vi "Scott -- strain -- plot staff V0.vi"(8 "error IN":errorcluster, 10 "plots control":cluster{"data string in":string, bool, bool}[](array[cluster]), 11 "data":dbl[][](array[numeric])) -> (0 "error out":errorcluster, 1 "Lockin 1 Graph":cluster{"X Data":dbl[], "Y Data":dbl[]}[](graph)=[{"X Data"=array[300 elements], "Y Data"=array[300 elements]}, {"X Data"=array[300 elements], "Y Data"=[0.34598, 0.34601, 0.34601, 0.34598, 0.34598, 0.34598, 0.34598, 0.34598, 0.34598, 0.34598, 0.34598, 0.34598, 0.34598, 0.345949, 0.34598, 0.34598, 0.34598, 0.34598, 0.34598, 0.34598, 0.34598, 0.34598, 0.34598, 0.34598, 0.34598, 0.34598, 0.34598, 0.34598, 0.34598, 0.34598, 0.34598, 0.34598, 0.34598, 0.34601, 0.34601, 0.34601, 0.34601, 0.34601, 0.34601, 0.34601, 0.34601, 0.34601, 0.34601, 0.34601, 0.34601, 0.34601, 0.34601, 0.346041, 0.346041, 0.346041, 0.346041, 0.346041, 0.346041, 0.346041, 0.346041, 0.346071, 0.346071, 0.346071, 0.346071, 0.346071, 0.346071, 0.346071, 0.346071, 0.346071, 0.346071, 0.346071, 0.346071, 0.346071, 0.346071, 0.346071, 0.346071, 0.346071, 0.346071, 0.346071, 0.346041, 0.346071, 0.346071, 0.346071, 0.346041, 0.346041, 0.346041, 0.346041, 0.346041, 0.34601, 0.346041, 0.346041, 0.34601, 0.34601, 0.34601, 0.34601, 0.34601, 0.34601, 0.34601, 0.34601, 0.34601, 0.34601, 0.34601, 0.34601, 0.34601, 0.34598, 0.34598, 0.34598, 0.34601, 0.34598, 0.34598, 0.34598, 0.34598, 0.34598, 0.34598, 0.34598, 0.34598, 0.34598, 0.34598, 0.34598, 0.34598, 0.34598, 0.34598, 0.34598, 0.34598, 0.34598, 0.34598, 0.34598, 0.34598, 0.34598, 0.34598, 0.34598, 0.34598, 0.34598, 0.34598, 0.34598, 0.34598, 0.34598, 0.34598, 0.34601, 0.34601, 0.34601, 0.34601, 0.34601, 0.34601, 0.34601, 0.34601, 0.34601, 0.34601, 0.34601, 0.34601, 0.34601, 0.346041, 0.346041, 0.34601, 0.34601, 0.346041, 0.346041, 0.346041, 0.346041, 0.346041, 0.346071, 0.346071, 0.346041, 0.346071, 0.346071, 0.346071, 0.346071, 0.346071, 0.346071, 0.346071, 0.346071, 0.346071, 0.346071, 0.346071, 0.346071, 0.346071, 0.346071, 0.346041, 0.346041, 0.346071, 0.346041, 0.346041, 0.346041, 0.346041, 0.346041, 0.346041, 0.34601, 0.346041, 0.346041, 0.34601, 0.34601, 0.34601, 0.34601, 0.34601, 0.34601, 0.34601, 0.34601, 0.34601, 0.34601, 0.34601, 0.34601, 0.34601, 0.34601, 0.34598, 0.34598, 0.34598, 0.34598, 0.34598, 0.34598, 0.34598, 0.34598, 0.34598, 0.34598, 0.34598, 0.34598, 0.34598, 0.34598, 0.34598, 0.34598, 0.34598, 0.345949, 0.34598, 0.34598, 0.34598, 0.34598, 0.34598, 0.34598, 0.34598, 0.34598, 0.34598, 0.34598, 0.34598, 0.34598, 0.34598, 0.34598, 0.34601, 0.34601, 0.34601, 0.34601, 0.34601, 0.34601, 0.34601, 0.34601, 0.34601, 0.34601, 0.34601, 0.34601, 0.34601, 0.34601, 0.34601, 0.34601, 0.34601, 0.346041, 0.346041, 0.346041, 0.346041, 0.346041, 0.346071, 0.346071, 0.346041, 0.346041, 0.346071, 0.346071, 0.346071, 0.346071, 0.346071, 0.346071, 0.346071, 0.346071, 0.346071, 0.346071, 0.346071, 0.346071, 0.346071, 0.346071, 0.346071, 0.346071, 0.346071, 0.346071, 0.346071, 0.346071, 0.346071, 0.346071, 0.346071, 0.346041, 0.346041, 0.346041, 0.346041, 0.346041, 0.34601, 0.346041, 0.346041, 0.34601, 0.34601, 0.34601, 0.34601, 0.34601, 0.34601, 0.34601, 0.34601, 0.34601, 0.34601, 0.34601, 0.34601, 0.34601]}, {"X Data"=array[300 elements], "Y Data"=array[300 elements]}, {"X Data"=array[300 elements], "Y Data"=[0.018135, 0.018139, 0.018133, 0.018133, 0.018137, 0.018135, 0.018133, 0.018133, 0.018131, 0.018129, 0.018129, 0.018127, 0.018131, 0.018131, 0.018127, 0.018127, 0.018127, 0.018125, 0.018127, 0.018127, 0.018123, 0.018129, 0.018131, 0.018127, 0.018135, 0.018139, 0.018139, 0.01814, 0.01814, 0.018137, 0.018131, 0.018131, 0.018127, 0.018137, 0.01814, 0.018139, 0.018135, 0.018133, 0.018139, 0.018135, 0.018139, 0.018144, 0.018142, 0.01814, 0.018144, 0.01815, 0.018144, 0.018146, 0.01814, 0.018139, 0.018135, 0.018129, 0.018129, 0.018135, 0.018142, 0.01814, 0.01814, 0.018142, 0.018146, 0.018144, 0.018144, 0.01815, 0.018144, 0.01814, 0.01814, 0.018137, 0.018137, 0.018137, 0.01814, 0.01814, 0.018137, 0.018131, 0.018131, 0.018137, 0.018137, 0.018144, 0.01814, 0.018131, 0.018131, 0.018129, 0.018131, 0.018139, 0.018148, 0.018144, 0.018139, 0.018133, 0.018131, 0.018133, 0.018127, 0.018129, 0.018119, 0.018123, 0.018125, 0.018127, 0.018133, 0.018133, 0.018131, 0.018129, 0.018131, 0.018133, 0.018129, 0.018129, 0.018131, 0.018133, 0.018127, 0.018123, 0.018121, 0.018125, 0.018127, 0.018131, 0.018129, 0.018127, 0.018127, 0.018127, 0.018129, 0.018123, 0.018127, 0.018125, 0.018116, 0.018116, 0.018127, 0.018127, 0.018123, 0.018121, 0.018125, 0.018127, 0.018127, 0.018127, 0.018135, 0.018135, 0.018129, 0.018131, 0.018125, 0.018118, 0.018121, 0.018135, 0.018139, 0.01814, 0.018146, 0.018142, 0.01814, 0.018137, 0.018127, 0.018127, 0.018135, 0.01814, 0.01814, 0.018137, 0.018127, 0.018133, 0.018137, 0.018142, 0.018142, 0.01814, 0.01814, 0.01814, 0.018142, 0.01814, 0.018135, 0.01814, 0.01814, 0.018135, 0.018139, 0.018139, 0.01814, 0.01814, 0.018146, 0.018146, 0.01814, 0.018144, 0.018146, 0.018144, 0.018139, 0.018139, 0.018135, 0.018137, 0.01814, 0.01814, 0.018139, 0.018131, 0.018139, 0.018139, 0.018133, 0.018135, 0.018129, 0.018131, 0.018137, 0.018133, 0.018135, 0.018139, 0.018139, 0.018137, 0.018133, 0.018129, 0.018129, 0.018125, 0.018129, 0.018135, 0.018133, 0.018135, 0.018125, 0.018127, 0.018123, 0.018125, 0.018127, 0.018127, 0.018125, 0.018125, 0.018125, 0.018125, 0.018127, 0.018127, 0.018133, 0.018129, 0.018129, 0.018127, 0.018123, 0.018131, 0.018129, 0.018129, 0.018133, 0.018131, 0.018137, 0.018137, 0.018135, 0.018135, 0.018129, 0.018133, 0.018137, 0.018135, 0.018131, 0.018129, 0.018131, 0.018135, 0.018139, 0.01814, 0.018139, 0.018139, 0.018129, 0.018131, 0.01814, 0.018127, 0.018131, 0.018133, 0.018129, 0.018131, 0.018137, 0.018131, 0.018135, 0.01814, 0.018139, 0.018135, 0.018135, 0.018133, 0.018137, 0.018139, 0.018137, 0.018133, 0.01814, 0.01814, 0.018133, 0.018133, 0.018133, 0.01814, 0.018146, 0.018148, 0.018142, 0.01814, 0.01814, 0.018135, 0.018131, 0.01814, 0.01814, 0.01814, 0.01814, 0.01814, 0.018135, 0.018133, 0.018139, 0.018133, 0.018129, 0.018135, 0.018133, 0.018135, 0.018135, 0.018135, 0.018137, 0.018135, 0.018135, 0.018135, 0.018131, 0.018131, 0.018125, 0.018125, 0.018129, 0.018129, 0.018127, 0.018125, 0.018121, 0.018118]}] caption="XY Graph")   [LabVIEW 2014]
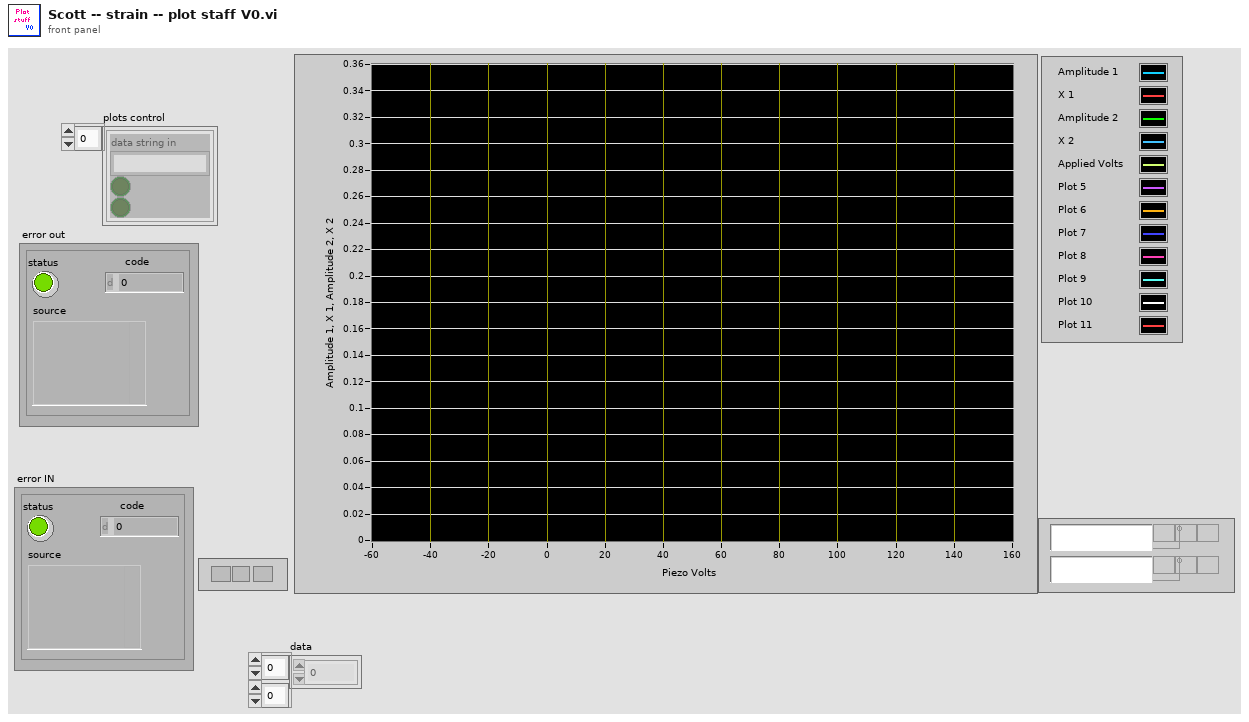
[diagram p1: front panel]
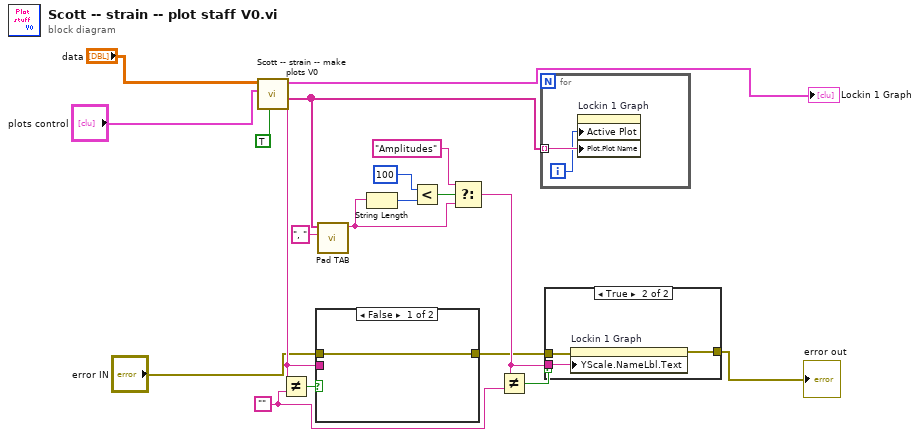
[diagram p0: block diagram]
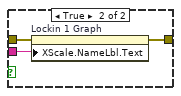
[diagram p3: hidden frame]
diagram:
  w9 = ""
  n1 = call "Scott -- strain -- make plots V0.vi"("transpose? (no:F)"=TRUE, "Channels to plot"="plots control", "Data"="data") -> ("Y-axis names"=w5:string[], "X-axis name"=w8:string, "Plots"=→"Lockin 1 Graph":cluster{"X Data":dbl[], "Y Data":dbl[]}[])  [unwired: 4 in, 2 out]
  n2 = Not Equal?(x=w8, y=w9) -> (x != y?=w11:bool)
  n3 = case shown="False" w11 {
    tunnel: w8 -> [_ w23]
    tunnel: "error IN" -> [w20 w22]
    tunnel: [w20 w21] -> w6
    frame False {
    }
    frame True {
      n4 = property on="Lockin 1 Graph" class="XYGraph (strict)"(error in=w22, "XScale.NameLbl.Text"=w23) -> (error out=w21:errorcluster)  [unwired: 1 in, 1 out]
    }
  }
  n5 = call "Pad TAB.vi"("Separator"=", ", "Input String Array"=w5) -> ("Output String"=w12:string)  [unwired: 9 in]
  n6 = String Length(string=w12) -> (length=w15:i32)
  n7 = Less?(x=100, y=w15) -> (x < y?=w16:bool)
  n8 = Select(t="Amplitudes", s=w16, f=w12) -> (s? t:f=w7:string)
  n9 = Not Equal?(x=w7, y=w9) -> (x != y?=w10:bool)
  n10 = for {
    tunnel: w5 -> [w25] mode=indexing
    i -> [w24]
    n11 = property on="Lockin 1 Graph" class="XYGraph (strict)"("Active Plot"=w24, "Plot.Plot Name"=w25) -> ()  [unwired: 2 in, 2 out]
  }
  n12 = case shown="True" w10 {
    tunnel: w7 -> [_ w29]
    tunnel: w6 -> [w26 w28]
    tunnel: [w26 w27] -> w3
    frame False {
    }
    frame True {
      n13 = property on="Lockin 1 Graph" class="XYGraph (strict)"(error in=w28, "YScale.NameLbl.Text"=w29) -> (error out=w27:errorcluster)  [unwired: 1 in, 1 out]
    }
  }
  "error out" <- w3
